vi "myCSVwrite.vi"(8 "错误输入（无错误）":errorcluster, 9 "字节流文件输入":refnum<file>, 10 "写表结果输入":dbl[][](array[numeric]), 11 "响应测试选项":u32(ring)=2 items=["仅测量信号", "单相扫频", "三相同步系扫频", "三相正负序扫频"]) -> (0 "错误输出":errorcluster, 1 "字节流文件输出":refnum<file>)   [LabVIEW 2024]
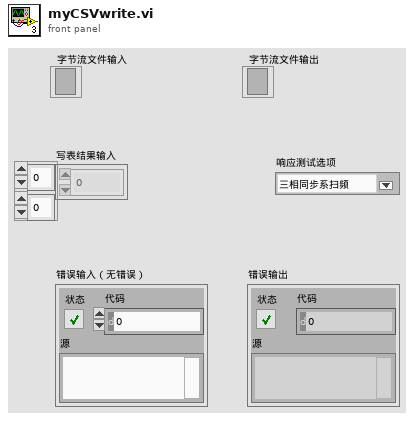
[diagram p1: front panel]
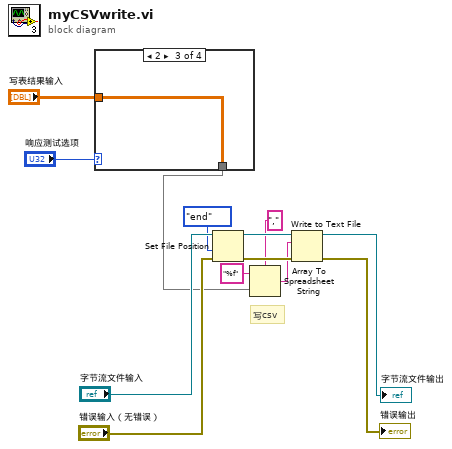
[diagram p0: block diagram]
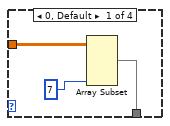
[diagram p2: hidden frame]
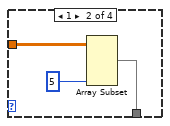
[diagram p3: hidden frame]
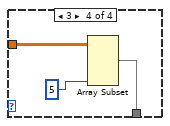
[diagram p4: hidden frame]
diagram:
  # "写csv"
  n1 = case shown="2" "响应测试选项" {
    tunnel: "写表结果输入" -> [w16 w19 w20 w22]
    tunnel: [w14 w17 w20 w21] -> w1
    frame 0, Default {
      n2 = Array Subset(array=w16, length (col)=7 ("长度")) -> (w14:dbl[][])  [unwired: 3 in]
    }
    frame 1 {
      n3 = Array Subset(array=w19, length (col)=5 ("长度")) -> (w17:dbl[][])  [unwired: 3 in]
    }
    frame 2 {
    }
    frame 3 {
      n4 = Array Subset(array=w22, length (col)=5 ("长度")) -> (w21:dbl[][])  [unwired: 3 in]
    }
  }
  n5 = Set File Position(refnum="字节流文件输入", from (0:start)=enum16{"start", "end", "current"}."end" ("自（0:起始）"), error in="错误输入（无错误）") -> (refnum out=w7:refnum<file>, error out=w8:errorcluster)  [unwired: 1 in]
  n6 = Array To Spreadsheet String(delimiter (Tab)="," ("name (excel)"), array=w1, 3:"%f" ("name (excel)")) -> (spreadsheet string=w6:string)
  n7 = Write to Text File(file (use dialog)=w7, text=w6, error in=w8) -> (refnum out=→"字节流文件输出":refnum<file>, error out=→"错误输出":errorcluster)  [unwired: 1 in, 1 out]
